vi "f_create file.vi"(11 "path":path=path "D:/Gantry_General/Main/ms_kao/gantry exericse/save test/002.txt") -> (3 "dup path":path=path "D:/Gantry_General/Main/ms_kao/gantry exericse/save test/002.txt")   [LabVIEW 2016]
panel:
  in  "operation (0:open)":T1(ring)=enum."create"
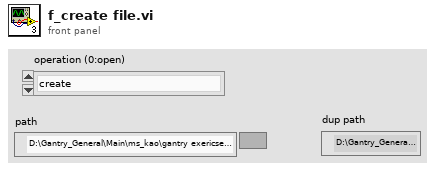
[diagram p1: front panel]
types:
  T1 = enum16{"open", "replace", "create", "open or create", "replace or create", "replace or create with confirmation"}
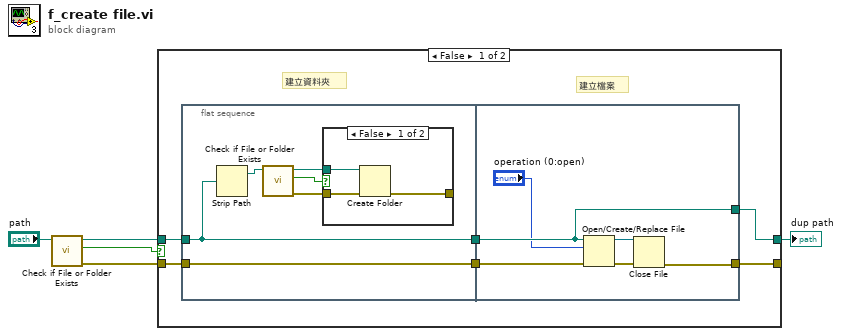
[diagram p0: block diagram]
diagram:
  n1 = call <vilib>:"Check if File or Folder Exists.vi"("path"="path") -> ("error out"=w2:errorcluster, "file or folder exists?"=w4:bool, "dup path"=w3:path)  [unwired: 8 in]
  n2 = case shown="False" w4 {
    tunnel: w3 -> [w10 w29]
    tunnel: w2 -> [w11 w28]
    tunnel: [w9 w28] -> _
    tunnel: [w8 w29] -> w1
    frame False {
      # "建立檔案"
      # "建立資料夾"
      n3 = flat-sequence {
        tunnel: w10 -> [w12]
        tunnel: w11 -> [w17]
        tunnel: [w17] -> w7
        tunnel: [w12] -> w6
        tunnel: [w22] -> w9
        tunnel: [w26] -> w8
        tunnel: w7 -> [w27]
        tunnel: w6 -> [w26]
        frame #0 {
          n4 = Strip Path(path=w12) -> (stripped path=w13:path)  [unwired: 1 out]
          n5 = call <vilib>:"Check if File or Folder Exists.vi"("path"=w13) -> ("error out"=w16:errorcluster, "file or folder exists?"=w14:bool, "dup path"=w15:path)  [unwired: 8 in]
          n6 = case shown="False" w14 {
            tunnel: w15 -> [w20 _]
            tunnel: [w19 w21] -> _
            tunnel: w16 -> [w18 w21]
            frame False {
              n7 = Create Folder(path (use dialog)=w20, error in=w18) -> (error out=w19:errorcluster)  [unwired: 1 in, 2 out]
            }
            frame True {
            }
          }
        }
        frame #1 {
          n8 = Open/Create/Replace File(file path (use dialog)=w26, error in=w27, operation (0:open)="operation (0:open)") -> (refnum out=w24:refnum<file>, error out=w23:errorcluster)  [unwired: 3 in, 1 out]
          n9 = Close File(refnum=w24, error in=w23) -> (error out=w22:errorcluster)  [unwired: 1 out]
        }
      }
    }
    frame True {
    }
  }
  "dup path" <- w1
